vi "_word.table.AppendNewLines.vi"(8 "error in (no error)":errorcluster, 9 "mode":enum16{"entire row", "entire column"}(ring), 10 "number":i32, 11 "table Refnum in":refnum<k7>) -> (0 "error out":errorcluster, 1 "Cluster":cluster{"x+1":i32, "x+1":i32}, 3 "table Refnum out":refnum<k7>)   [LabVIEW 2018, in "WordReportGeneration.lvlib"]
uses:
  WordReportGeneration.lvlib
  <vilib>/Utility/NIReport.llb/NI_ReportGenerationCore.lvlib
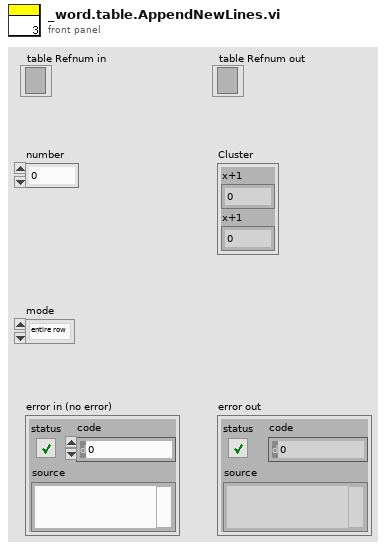
[diagram p1: front panel]
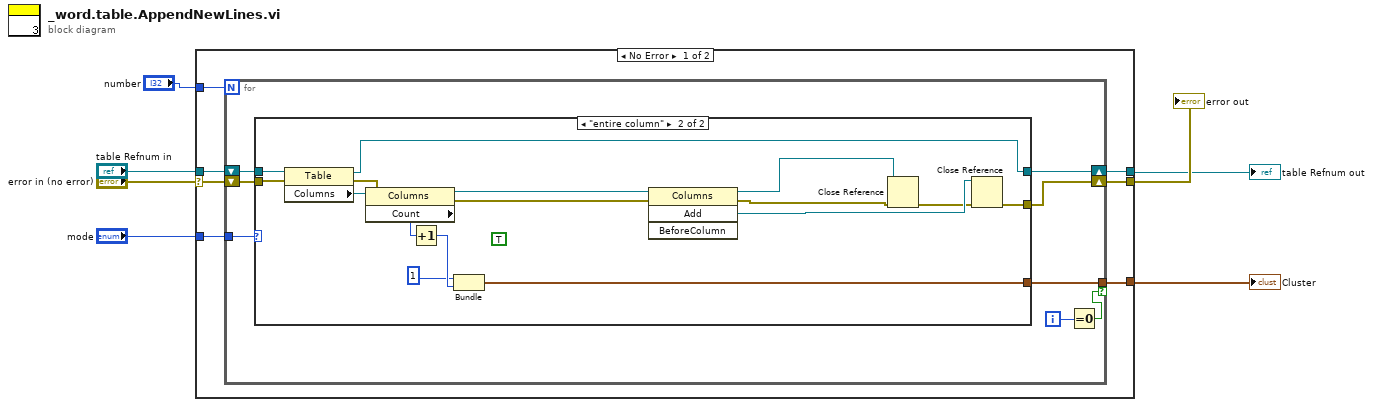
[diagram p0: block diagram]
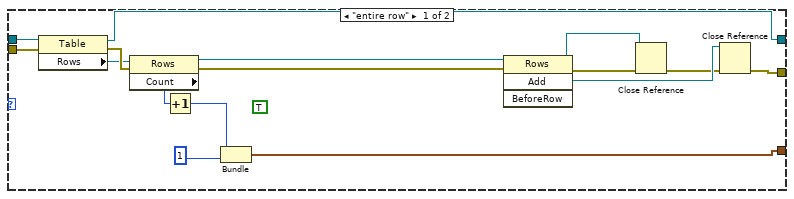
[diagram p2: hidden frame]
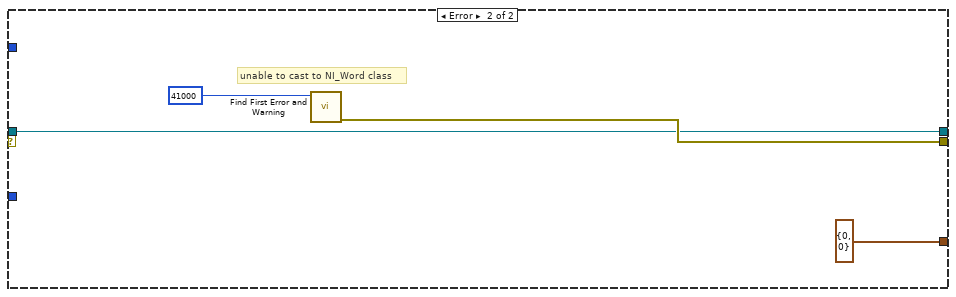
[diagram p3: hidden frame]
diagram:
  n1 = case shown="No Error" "error in (no error)" {
    selector: "error in (no error)" -> [w11 _]
    tunnel: "mode" -> [w14 _]
    tunnel: [w13 w57] -> w6
    tunnel: "table Refnum in" -> [w12 w56]
    tunnel: [w10 w56] -> w3
    tunnel: "number" -> [w9 _]
    tunnel: [w8 cluster{"x+1":i32, i32} {"x+1"=0, 0}] -> w1
    frame No Error {
      n2 = for {
        N: w9 -> [_]
        tunnel: w14 -> [w22]
        shift-right: [w18] -> w10
        shift-left: w12 -> [w20]
        shift-right: [w21] -> w13
        shift-left: w11 -> [w19]
        tunnel: [w17] -> w8 if=w15
        i -> [w16]
        n3 = case shown="\"entire column\"" w22 {
          tunnel: w20 -> [w38 w46]
          tunnel: w19 -> [w37 w45]
          tunnel: [w35 w44] -> w21
          tunnel: [w26 w42] -> w18
          tunnel: [w23 w40] -> w17
          frame "entire row" {
            (unwired) TRUE
            n4 = property class="Table"(reference=w38, error in=w37) -> (reference out=w26:refnum<k7>, error out=w33:errorcluster, "Rows"=w32:refnum<k7>)
            n5 = property class="Rows"(reference=w32, error in=w33) -> (reference out=w30:refnum<k7>, error out=w31:errorcluster, "Count"=w29:i32)
            n6 = Increment(x=w29) -> (x+1=w24:i32)
            n7 = Bundle(w24, "x+1"=1) -> (w23:cluster{i32, "x+1":i32})  [unwired: 1 in]
            n8 = invoke class="Rows" method="Add"(reference=w30, error in=w31) -> (reference out=w28:refnum<k7>, error out=w36:errorcluster, "Add"=w34:refnum<k7>)  [unwired: 2 in, 1 out]
            n9 = Close Reference(reference=w28, error in (no error)=w36) -> (error out=w27:errorcluster)
            n10 = Close Reference(reference=w34, error in (no error)=w27) -> (error out=w35:errorcluster)
          }
          frame "entire column" {
            (unwired) TRUE
            n11 = property class="Table"(reference=w46, error in=w45) -> (reference out=w42:refnum<k7>, error out=w51:errorcluster, "Columns"=w50:refnum<k7>)
            n12 = property class="Columns"(reference=w50, error in=w51) -> (reference out=w48:refnum<k7>, error out=w49:errorcluster, "Count"=w47:i32)
            n13 = Increment(x=w47) -> (x+1=w41:i32)
            n14 = Bundle("x+1"=1, w41) -> (w40:cluster{"x+1":i32, i32})  [unwired: 1 in]
            n15 = invoke class="Columns" method="Add"(reference=w48, error in=w49) -> (reference out=w53:refnum<k7>, error out=w54:errorcluster, "Add"=w52:refnum<k7>)  [unwired: 2 in, 1 out]
            n16 = Close Reference(reference=w53, error in (no error)=w54) -> (error out=w43:errorcluster)
            n17 = Close Reference(reference=w52, error in (no error)=w43) -> (error out=w44:errorcluster)
          }
        }
        n18 = Equal To 0?(x=w16) -> (x = 0?=w15:bool)
      }
    }
    frame Error {
      # "unable to cast to NI_Word class"
      n19 = call <vilib>:"Find First Error and Warning.vi"("error code"=41000) -> ("error out"=w57:errorcluster)  [unwired: 2 in, 4 out]
    }
  }
  "error out" <- w6
  "table Refnum out" <- w3
  "Cluster" <- w1
